vi "Notify Monitor.vi"(8 "error in":errorcluster, 11 "Monitored Actor in":refnum<class "Monitored Actor.lvclass">) -> (0 "error out":errorcluster, 3 "Monitored Actor out":refnum<class "Monitored Actor.lvclass">)   [LabVIEW 2023, in "Monitored Actor.lvlib" / "Monitored Actor.lvclass"]
doc: "Notifies the actor monitor that a new actor has spawned\n\nCopyright: MGI 2016\nAuthor: Derek Trepanier"
uses:
  Monitored Actor.lvclass
  C:/Users/Public/Documents/Development/builds/Engine/Actor Framework.lvlibp/1abvi3w/vi.lib/ActorFramework/Actor/Actor.lvclass
  Monitored Actor.lvclass/Monitored Actor.ctl
  builds/Engine/Actor Framework.lvlibp/1abvi3w/vi.lib/ActorFramework/Actor/Read Actor Label.vi
  builds/Engine/Actor Framework.lvlibp/1abvi3w/vi.lib/ActorFramework/Actor/Write Actor Label.vi
  Actor Monitor/Actor Monitor Messages/Actor Launched Msg/Actor Launched Msg.lvclass
  Actor Monitor/Actor Monitor Messages/Update Label Msg/Update Label Msg.lvclass
  builds/Engine/Actor Framework.lvlibp/1abvi3w/vi.lib/ActorFramework/Message Enqueuer/Message Enqueuer.lvclass
  builds/Engine/Actor Framework.lvlibp/1abvi3w/vi.lib/ActorFramework/Actor/Actor.lvclass
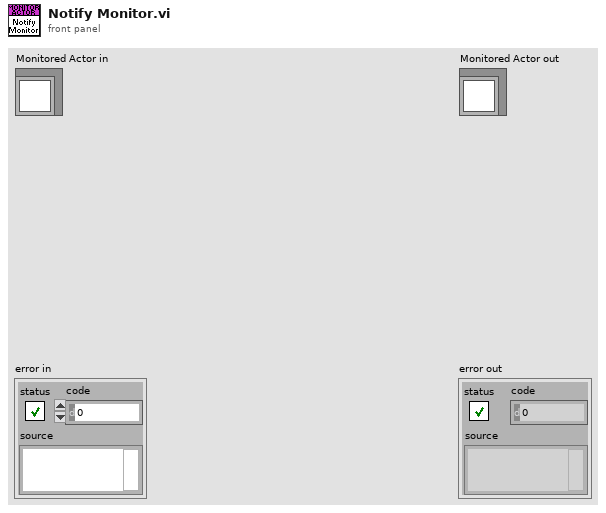
[diagram p1: front panel]
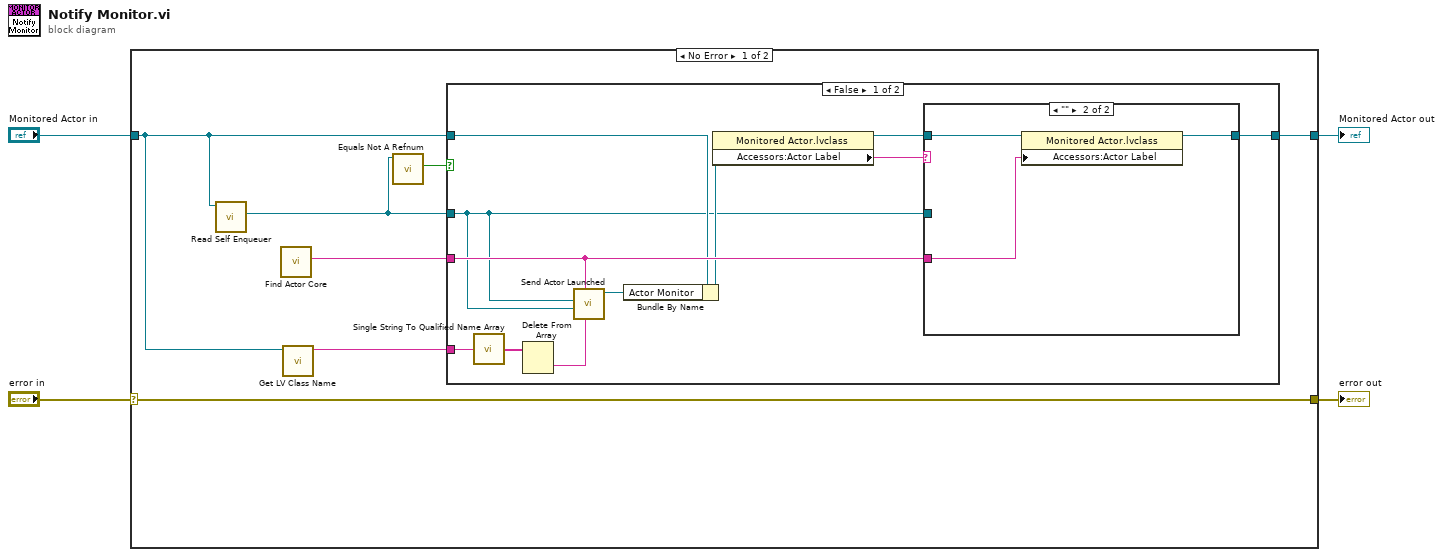
[diagram p0: block diagram]
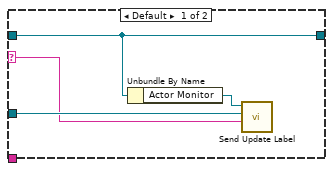
[diagram p2: hidden frame]
diagram:
  n1 = case shown="No Error" "error in" {
    selector: "error in" -> [w7 w32]
    tunnel: [w7 w32] -> w3
    tunnel: [w11 w31] -> w1
    tunnel: "Monitored Actor in" -> [w6 w31]
    frame No Error {
      n2 = call "Read Self Enqueuer.vi"("Actor"=w6) -> ("Self Enqueuer"=w5:refnum<class "Message Enqueuer.lvclass">)  [unwired: 10 in]
      n3 = call "Find Actor Core.vi"() -> ("Actor Core VI Name"=w10:string)  [unwired: 10 in, 1 out]
      n4 = call <vilib>:"Get LV Class Name.vi"("object"=w6) -> ("class name"=w9:string)  [unwired: 9 in, 1 out]
      n5 = call "Equals Not A Refnum.vi"("Message Enqueuer"=w5) -> ("Not a refnum?"=w8:bool)  [unwired: 10 in]
      n6 = case shown="False" w8 {
        tunnel: [w22 w30] -> w11
        tunnel: w10 -> [w21 _]
        tunnel: w6 -> [w20 w30]
        tunnel: w9 -> [w19 _]
        tunnel: w5 -> [w14 _]
        frame False {
          n7 = call <vilib>:"Single String To Qualified Name Array.vi"("Fully Qualified String"=w19) -> ("Fully Qualified Array"=w18:string[])
          n8 = Delete From Array(array=w18) -> (deleted portion=w17:string)  [unwired: 2 in, 1 out]
          n9 = call "Send Actor Launched.vi"("Actor Type"=w17, "Actor Core VI"=w21, "Actor's Caller Q"=w14, "Actor's Self Q"=w14) -> ("Message Enqueuer out"=w15:refnum<class "Message Enqueuer.lvclass">)  [unwired: 6 in, 1 out]
          n10 = Bundle By Name(cluster=w20, "Actor Monitor"=w15) -> (w16:refnum<class "Monitored Actor.lvclass">)
          n11 = property class="Monitored Actor.lvclass"(reference=w16) -> (reference out=w13:refnum<class "Monitored Actor.lvclass">, "Accessors:Actor Label"=w12:string)  [unwired: 1 in, 1 out]
          n12 = case shown="\"\"" w12 {
            selector: w12 -> [w25 _]
            tunnel: w13 -> [w24 w28]
            tunnel: w14 -> [w26 _]
            tunnel: [w24 w29] -> w22
            tunnel: w21 -> [_ w27]
            frame Default {
              n13 = Unbundle By Name(w24) -> ("Actor Monitor"=w23:refnum<class "Message Enqueuer.lvclass">)
              n14 = call "Send Update Label.vi"("Actor's Label"=w25, "Actor's Self Q"=w26, "Message Enqueuer in"=w23) -> ()  [unwired: 7 in, 2 out]
            }
            frame "" {
              n15 = property class="Monitored Actor.lvclass"(reference=w28, "Accessors:Actor Label"=w27) -> (reference out=w29:refnum<class "Monitored Actor.lvclass">)  [unwired: 1 in, 1 out]
            }
          }
        }
        frame True {
        }
      }
    }
    frame Error {
    }
  }
  "error out" <- w3
  "Monitored Actor out" <- w1
